vi "vi.GetArrayType.vi"(11 "VarArray in":variant) -> (4 "Dims":u32, 8 "type":T1(ring), 15 "VarArray out":variant)   [LabVIEW 2014, in "GLue.lvlib" / "class.GLue.lvclass"]
uses:
  class.GLue.lvclass
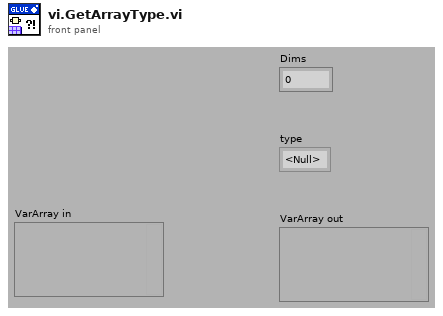
[diagram p1: front panel]
types:
  T1 = enum8{"<Null>", "I8", "I16", "I32", "I64", "U8", "U16", "U32", "U64", "SGL", "DBL", "EXT", "CSG", "CDB", "CXT", "0x0F", "0x10", "0x11", "0x12", "0x13", "0x14", "Enum U8", "Enum U16", "Enum U32", "Enum U64", "SGL PQ", "DBL PQ", "EXT PQ", "CSG PQ", "CDB PQ", "CXT PQ", "0x1F", "0x20", "Boolean", "0x22", "0x23", "0x24", "0x25", "0x26", "0x27", "0x28", "0x29", "0x2A", "0x2B", "0x2C", "0x2D", "0x2E", "0x2F", "String", "0x31", "Path", "Pict", "0x34", "0x35", "0x36", "DAQ", "0x38", "0x39", "0x3A", "0x3B", "0x3C", "0x3D", "0x3E", "0x3F", "Array", "0x41", "0x42", "0x43", "0x44", "0x45", "0x46", "0x47", "0x48", "0x49", "0x4A", "0x4B", "0x4C", "0x4D", "0x4E", "0x4F", "Cluster", "0x51", "0x52", "Variant", "Waveform", "0x55", "0x56", "0x57", "0x58", "0x59", "0x5A", "0x5B", "0x5C", "0x5D", "0x5E", "0x5F", "0x60", "0x61", "0x62", "0x63", "0x64", "0x65", "0x66", "0x67", "0x68", "0x69", "0x6A", "0x6B", "0x6C", "0x6D", "0x6E", "0x6F", "Refnum"}
  T2 = cluster{"length":u16, "private":u8, "type":enum8{"<Null>", "I8", "I16", "I32", "I64", "U8", "U16", "U32", "U64", "SGL", "DBL", "EXT", "CSG", "CDB", "CXT", "0x0F", "0x10", "0x11", "0x12", "0x13", "0x14", "Enum U8", "Enum U16", "Enum U32", "Enum U64", "SGL PQ", "DBL PQ", "EXT PQ", "CSG PQ", "CDB PQ", "CXT PQ", "0x1F", "0x20", "Boolean", "0x22", "0x23", "0x24", "0x25", "0x26", "0x27", "0x28", "0x29", "0x2A", "0x2B", "0x2C", "0x2D", "0x2E", "0x2F", "String", "0x31", "Path", "Pict", "0x34", "0x35", "0x36", "DAQ", "0x38", "0x39", "0x3A", "0x3B", "0x3C", "0x3D", "0x3E", "0x3F", "Array", "0x41", "0x42", "0x43", "0x44", "0x45", "0x46", "0x47", "0x48", "0x49", "0x4A", "0x4B", "0x4C", "0x4D", "0x4E", "0x4F", "Cluster", "0x51", "0x52", "Variant", "Waveform", "0x55", "0x56", "0x57", "0x58", "0x59", "0x5A", "0x5B", "0x5C", "0x5D", "0x5E", "0x5F", "0x60", "0x61", "0x62", "0x63", "0x64", "0x65", "0x66", "0x67", "0x68", "0x69", "0x6A", "0x6B", "0x6C", "0x6D", "0x6E", "0x6F", "Refnum"}, "# elements":u16}
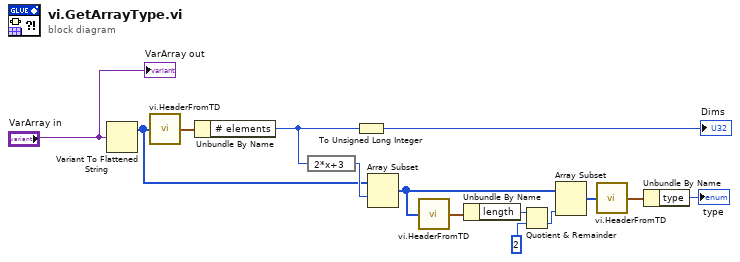
[diagram p0: block diagram]
diagram:
  n1 = Variant To Flattened String(Variant="VarArray in") -> (1:w7:i16[])  [unwired: 1 out]
  n2 = call "vi.HeaderFromTD.vi"("Type Descriptor"=w7) -> ("Type Descriptor Header"=w14:T2)  [unwired: 4 in]
  n3 = Unbundle By Name(w14) -> ("# elements"=w5:u16)
  n4 = expression code="2*x+3"(w5) -> (w10:u16)
  n5 = To Unsigned Long Integer(number=w5) -> (unsigned 32bit integer=→"Dims":u32)
  n6 = Array Subset(array=w7, index=w10) -> (w8:i16[])  [unwired: 1 in]
  n7 = call "vi.HeaderFromTD.vi"("Type Descriptor"=w8) -> ("Type Descriptor Header"=w9:T2)  [unwired: 4 in]
  n8 = Unbundle By Name(w9) -> ("length"=w11:u16)
  n9 = Quotient & Remainder(x=w11, y=u16 2) -> (floor(x/y)=w13:u16)  [unwired: 1 out]
  n10 = Array Subset(array=w8, length=w13) -> (w6:i16[])  [unwired: 1 in]
  n11 = call "vi.HeaderFromTD.vi"("Type Descriptor"=w6) -> ("Type Descriptor Header"=w2:T2)  [unwired: 4 in]
  n12 = Unbundle By Name(w2) -> ("type"=→"type":T1)
  "VarArray out" <- "VarArray in"
